vi "VNA Initial.vi"(9 "Cal File Name Path":string="D:\\CALFILES\\27G.csa", 10 "VNA Model:":enum16{"E5071C", "N5230A(C)", "N5224A"}(ring)=enum."N5224A", 11 "VNA VISA":refnum<visa-resource-name>="TCPIP0::A-N5224A-41544.local::hislip0::INSTR") -> (3 "Connect?":bool=TRUE)   [LabVIEW 2011]
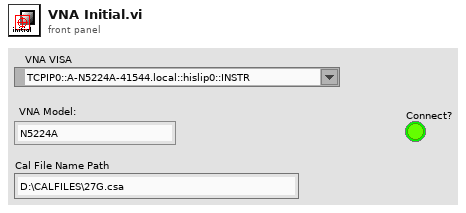
[diagram p1: front panel]
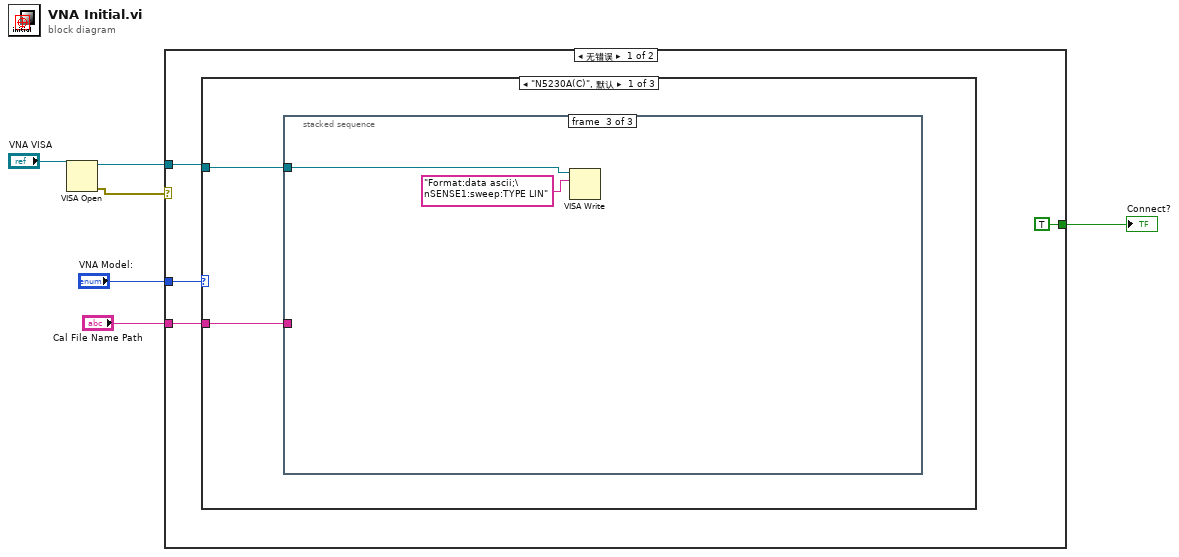
[diagram p0: block diagram]
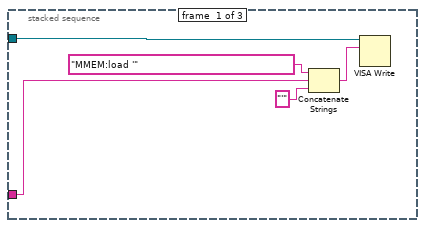
[diagram p2: hidden frame]
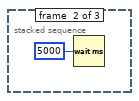
[diagram p3: hidden frame]
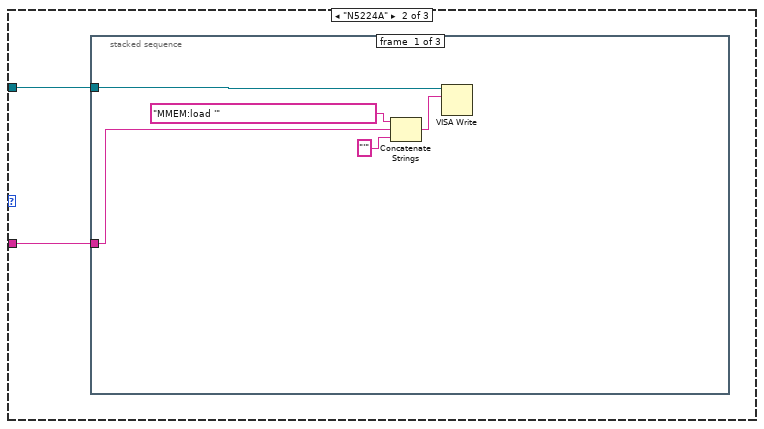
[diagram p4: hidden frame]
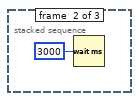
[diagram p5: hidden frame]
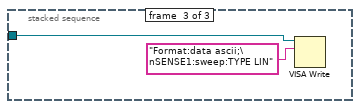
[diagram p6: hidden frame]
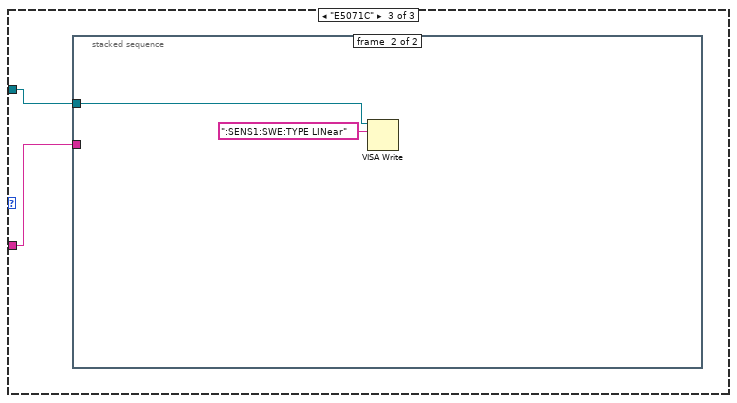
[diagram p7: hidden frame]
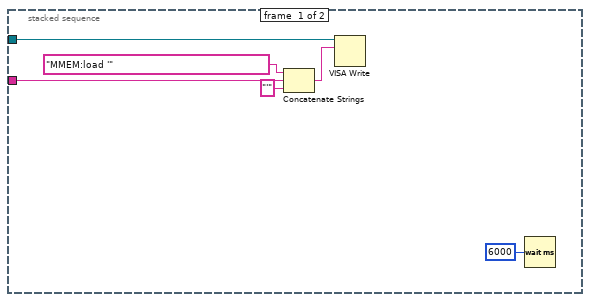
[diagram p8: hidden frame]
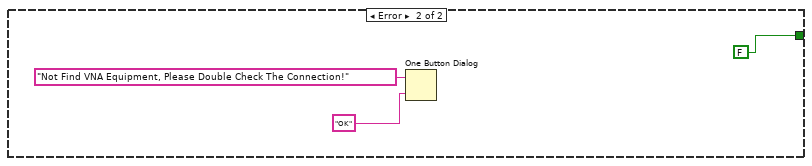
[diagram p9: hidden frame]
diagram:
  n1 = VISA Open(VISA resource name="VNA VISA") -> (VISA resource name=w4:refnum<visa-resource-name>, error out=w2:errorcluster)  [unwired: 4 in]
  n2 = case shown="无错误" w2 {
    tunnel: "VNA Model:" -> [w10 _]
    tunnel: w4 -> [w9 _]
    tunnel: "Cal File Name Path" -> [w8 _]
    tunnel: [TRUE FALSE] -> w1
    frame No Error {
      n3 = case shown="\"N5230A(C)\", 默认" w10 {
        tunnel: w9 -> [w12 w22 w32]
        tunnel: w8 -> [w11 w21 w31]
        frame "N5230A(C)", Default {
          n4 = stacked-sequence {
            tunnel: w12 -> [w17 _ w19]
            tunnel: w11 -> [w14 _ _]
            frame #0 {
              n5 = Concatenate Strings("MMEM:load '" ("write buffer"), w14, "'" ("字符串")) -> (w15:string)
              n6 = VISA Write(VISA resource name=w17, write buffer=w15) -> ()  [unwired: 1 in, 3 out]
            }
            frame #1 {
              n7 = Wait (ms)(milliseconds to wait=u32 5000) -> ()  [unwired: 1 out]
            }
            frame #2 {
              n8 = VISA Write(VISA resource name=w19, write buffer="Format:data ascii;\nSENSE1:sweep:TYPE LIN") -> ()  [unwired: 1 in, 3 out]
            }
          }
        }
        frame "N5224A" {
          n9 = stacked-sequence {
            tunnel: w22 -> [w27 _ w29]
            tunnel: w21 -> [w24 _ _]
            frame #0 {
              n10 = Concatenate Strings("MMEM:load '" ("write buffer"), w24, "'" ("字符串")) -> (w25:string)
              n11 = VISA Write(VISA resource name=w27, write buffer=w25) -> ()  [unwired: 1 in, 3 out]
            }
            frame #1 {
              n12 = Wait (ms)(milliseconds to wait=u32 3000) -> ()  [unwired: 1 out]
            }
            frame #2 {
              n13 = VISA Write(VISA resource name=w29, write buffer="Format:data ascii;\nSENSE1:sweep:TYPE LIN") -> ()  [unwired: 1 in, 3 out]
            }
          }
        }
        frame "E5071C" {
          n14 = stacked-sequence {
            tunnel: w32 -> [w35 w39]
            tunnel: w31 -> [w34 _]
            frame #0 {
              n15 = Concatenate Strings("MMEM:load '" ("write buffer"), w34, "'" ("字符串")) -> (w37:string)
              n16 = VISA Write(VISA resource name=w35, write buffer=w37) -> ()  [unwired: 1 in, 3 out]
              n17 = Wait (ms)(milliseconds to wait=u32 6000 ("等待时间（毫秒）")) -> ()  [unwired: 1 out]
            }
            frame #1 {
              n18 = VISA Write(VISA resource name=w39, write buffer=":SENS1:SWE:TYPE LINear") -> ()  [unwired: 1 in, 3 out]
            }
          }
        }
      }
    }
    frame Error {
      n19 = One Button Dialog(message="Not Find VNA Equipment, Please Double Check The Connection!" ("消息"), button name ("OK")="OK" ("按钮名称（“确定”）")) -> ()  [unwired: 1 out]
    }
  }
  "Connect?" <- w1
